vi "Generate String Array.vi"(5 "Shuffle?":bool, 7 "Contain Duplicates?":bool, 8 "Array Size":i32, 9 "Generate Methods":string[](array[combo]), 10 "m":i32, 11 "Format String":string="%s") -> ()   [LabVIEW 2021, in "EDT Array.lvlib"]
uses:
  EDT Array.lvlib
  49ae8d3a-0f37-470e-9090-99ed19fa0c2f.vi
panel:
  out "size(s)":i32
  out "C(n,m) Items":i32[](array[numeric])
  in  "n":i32
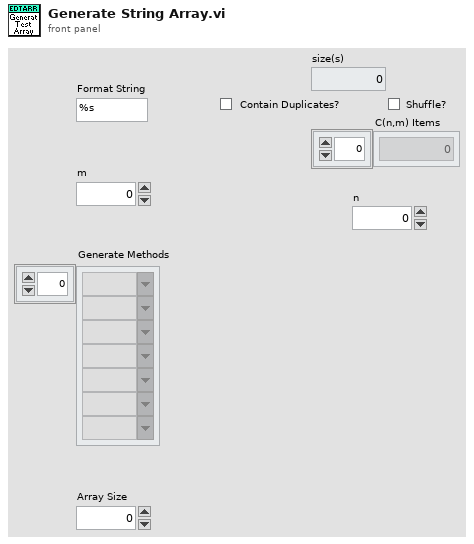
[diagram p1: front panel]
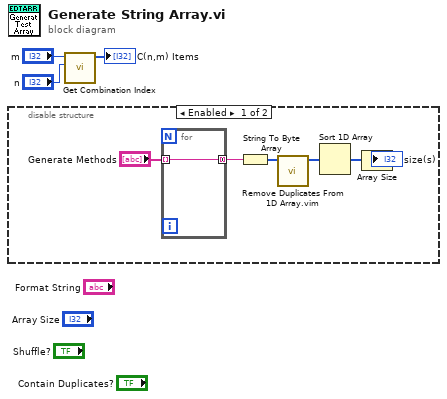
[diagram p0: block diagram]
diagram:
  n1 = disable-structure shown="Enabled" {
    frame Enabled {
      n2 = for {
        tunnel: "Generate Methods" -> [w10] mode=indexing
        tunnel: [w10] -> w8 mode=concatenating
      }
      n3 = String To Byte Array(string=w8) -> (unsigned byte array=w7:u8[])
      n4 = call "Remove Duplicates From 1D Array.vim"("array"=w7) -> ("array with duplicates removed"=w6:u8[])  [unwired: 10 in]
      n5 = Sort 1D Array(array=w6) -> (sorted array=w5:u8[])
      n6 = Array Size(array=w5) -> (size(s)=→"size(s)":i32)
    }
    frame Disabled {
    }
  }
  n7 = call "Get Combination Index.vi"("n"="n", "m"="m") -> ("C(n,m) Items"=→"C(n,m) Items":i32[])  [unwired: 8 in, 1 out]
